vi "Nick FP.vi"() -> ()   [LabVIEW 2013]
uses:
  cPAS/Interface/CRDS/Controls/Ringdown Xctl/Ringdown.xctl
  Reusable/CRDS/Data/Cell/extparam.ctl
  cPAS/UI/CRDS/Subject/CRD Subject.lvclass
  Timothy/File Observer/Tim File Observer.lvclass
  Reusable/Observer/Observer.lvclass/Observer.ctl
  Reusable/File IO/Class/File Observer.lvclass/File Observer.ctl
  Reusable/CRDS/Data/Main/CRDS Data.lvclass
  Reusable/Data/Data.lvclass
  Reusable/CRDS/Data/Cell/CRDS Cell Data.lvclass/CRDS Cell Data.ctl
  Reusable/Observer/Data Subject.lvclass/Data Subject.ctl
  Reusable/Observer/Accessors/Read Observer Refs.vi
  Reusable/Observer/Accessors/Read DVR.vi
  Reusable/CRDS/Data/Cell/Read extParam.vi
  Reusable/File IO/Class/Write Write.vi
  Reusable/Observer/Write Data Queue.vi
  Reusable/File IO/Class/Accessors/Write File Ext.vi
  Reusable/File IO/Class/Accessors/Write File Prefix.vi
  Reusable/File IO/Class/Accessors/Write Max Size.vi
  Reusable/File IO/Class/Accessors/Write Top Data Path.vi
  <vilib>/addons/Digital Filter Design/Process.llb/DFD Filtering (Array).vi
  Reusable/CRDS/Data/Main/Read CellData.vi
  Reusable/Data/Read measTime.vi
  Reusable/CRDS/Data/Cell/Read Ringdowns.vi
  Reusable/Observer/Data Subject.lvclass
  Reusable/File IO/Class/File Observer.lvclass
  Reusable/Observer/Observer.lvclass
  Reusable/CRDS/Data/Cell/CRDS Cell Data.lvclass
  <vilib>/addons/Digital Filter Design/NI_DigFilterLicensed.lvlib
panel:
  out "Waveform Graph":dbl[][](graph)
  out "Ext Data":T1[](array[typedef])
  out "tau":T2(graph)
  in  "Write?":bool
  in  "SamplesPerCycle":u16=100
  in  "PointsPerCycle":u16=1000
  out "Time":timestamp format="%<%H:%M:%S%3u>T"
  out "Ringdown":i16[][][](xcontrol)
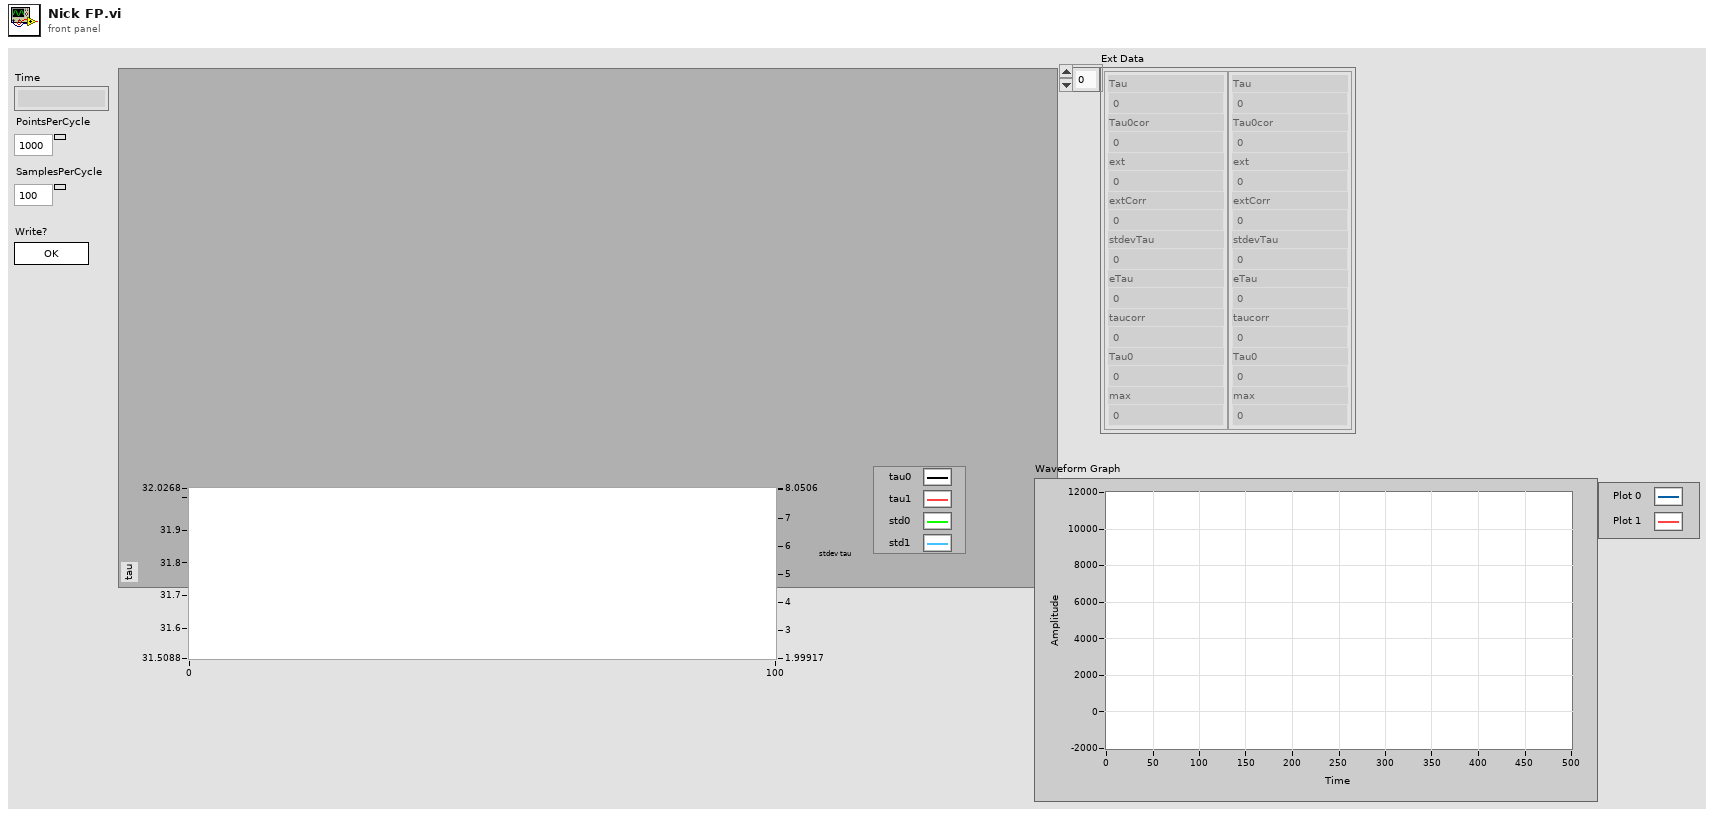
[diagram p1: front panel]
types:
  T1 = typedef "extparam.ctl" = cluster{"Tau":sgl, "Tau0cor":sgl, "ext":sgl, "extCorr":sgl, "stdevTau":sgl, "eTau":sgl, "taucorr":sgl, "Tau0":sgl, "max":sgl}
  T2 = cluster{"Tau":sgl, "Tau":sgl, "stdevTau":sgl, "stdevTau":sgl}
  T3 = typedef "NI_DigFilterLicensed.lvlib/DFD Filter Obj.ctl" = cluster{"mSRate_Fs":dbl, "mSRate_Version":string, "mSRate_Comments":string, "mSRate_OrgCoef":T4, "mSRate_CurCoef":T4, "mSRate_Quantized?":bool, "mSRate_QCoef":T4, "mSRate_QSettings":T6[], "mSRate_Order":i32, "mSRate_Scaling":cluster{"mSRate_ScaleByPowerOf2?":bool, "mSRate_ScaleType":T8}}
  T4 = typedef "NI_DigFilterLicensed.lvlib/DFD Filter Coef.ctl" = cluster{"type":T5, "gain":dbl, "coef a (k)":dbl[], "coef b (v)":dbl[]}
  T5 = typedef "NI_DigFilterLicensed.lvlib/DFD Filter Structure Type Selector.ctl" = enum16{"Undefined", "FIR Direct Form", "FIR Direct Form Transposed", "FIR Symmetric", "FIR Antisymmetric", "IIR Direct Form I", "IIR Direct Form I Transposed", "IIR Direct Form II", "IIR Direct Form II Transposed", "IIR Cascaded Second Order Sections Form I", "IIR Cascaded Second Order Sections Form I Transposed", "IIR Cascaded Second Order Sections Form II", "IIR Cascaded Second Order Sections Form II Transposed", "Lattice Allpass (basic sections)", "Lattice Allpass (one multiplier sections)", "Lattice Allpass (normalized sections)", "Lattice AR (basic sections)", "Lattice AR (one multiplier sections)", "Lattice AR (normalized sections)", "Lattice MA (minimum phase)", "Lattice MA (maximum phase)", "Lattice ARMA (basic sections)", "Lattice ARMA (one multiplier sections)", "Lattice ARMA (normalized sections)"}
  T6 = typedef "NI_DigFilterLicensed.lvlib/dfd_Internal Quantization Settings.ctl" = cluster{"source":T7, "wl":i16, "iwl":i16, "overflow mode":enum16{"Saturation", "Wrap"}, "rounding mode":enum16{"Nearest", "Truncation"}, "signed?":bool}
  T7 = typedef "NI_DigFilterLicensed.lvlib/dfd_Internal Quantization Srcs.ctl" = u16
  T8 = typedef "NI_DigFilterLicensed.lvlib/DFD Coef Norm Type.ctl" = enum16{"No Norm", "Time Domain 1-Norm", "Time Domain 2-Norm", "Time Domain Inf-Norm"}
  T9 = cluster{sgl, sgl, "stdevTau":sgl, "stdevTau":sgl}
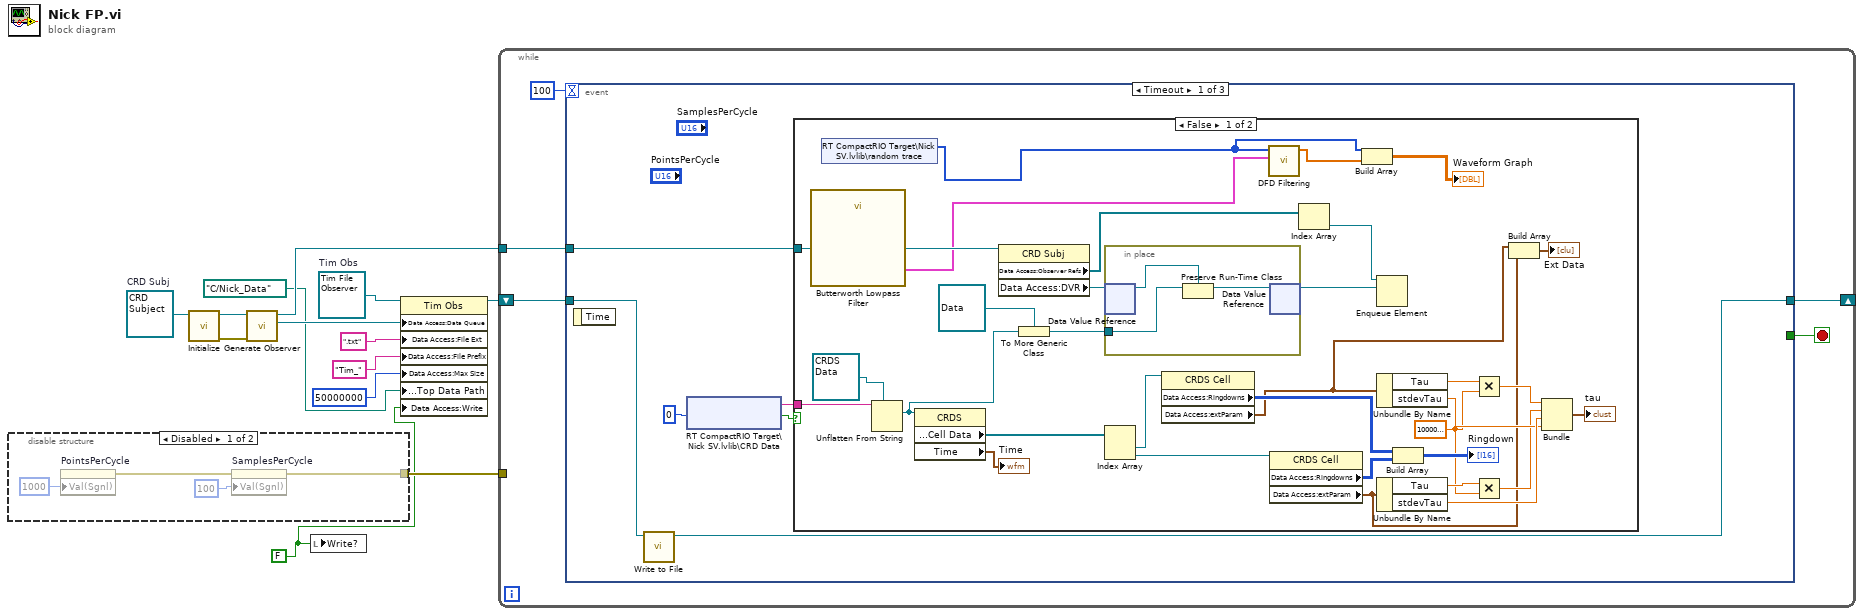
[diagram p0: block diagram]
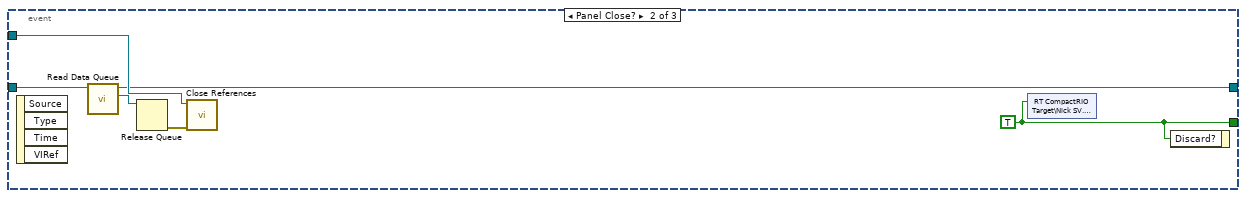
[diagram p4: hidden frame]
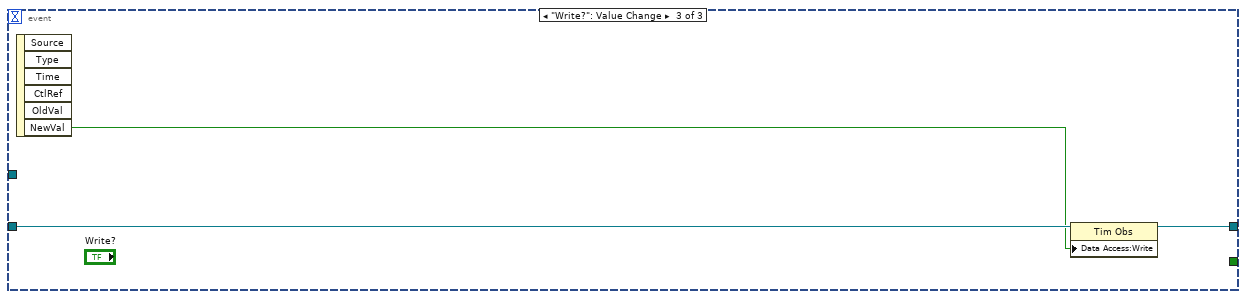
[diagram p5: hidden frame]
diagram:
  w2 = refnum<class "Tim File Observer.lvclass"> refnum  # Tim Obs
  w1 = FALSE ("Write")
  w12 = refnum<class "CRD Subject.lvclass"> refnum  # CRD Subj
  n1 = disable-structure shown="Disabled" {
    disable-tunnel: [w14 _] -> w13
    frame Disabled {
      n2 = property on="PointsPerCycle" class="DigNum (strict)"("Val(Sgnl)"=u16 1000 ("Value (Signaling)")) -> (error out=w15:errorcluster)  [unwired: 2 in, 1 out]
      n3 = property on="SamplesPerCycle" class="DigNum (strict)"(error in=w15, "Val(Sgnl)"=u16 100 ("Value (Signaling)")) -> (error out=w14:errorcluster)  [unwired: 1 in, 1 out]
    }
    frame Enabled {
    }
  }
  n4 = call-dynamic "Initialize.vi"("CRD Subject in"=w12) -> ("error out"=w10:errorcluster, "CRD Subject out"=w11:refnum<class "CRD Subject.lvclass">)  [unwired: 8 in, 1 out]
  n5 = call "Generate Observer.vi"("error in"=w10, "Data Subject in"=w11) -> ("Observer"=w9:refnum<queue>, "Data Subject out"=w8:refnum<class "CRD Subject.lvclass">)  [unwired: 7 in, 1 out]
  n6 = local write "Write?"(w1) -> ()
  n7 = property class="Tim Obs"(reference=w2, "Data Access:Data Queue"=w9, "Data Access:File Ext"=".txt" ("File Ext"), "Data Access:File Prefix"="Tim_" ("File Prefix"), "Data Access:Max Size"=i64 50000000 ("Max Size"), "Data Access:Top Data Path"=path "C:/Nick_Data" ("Top Data Path"), "Data Access:Write"=w1) -> (reference out=w3:refnum<class "Tim File Observer.lvclass">)  [unwired: 1 in, 1 out]
  n8 = while {
    tunnel: w13 -> [_]
    tunnel: w8 -> [w20]
    shift-right: [w18] -> _
    shift-left: w3 -> [w19]
    stop <- w22 stop-if-true
    n9 = event shown="[0] Timeout" {
      selector: _ -> [_ _ _]
      dyn-events: _ -> [_ _ _]
      timeout: 100 -> [_ _ _]
      tunnel: [_ w69 _] -> w22
      tunnel: w20 -> [w25 w68 _]
      tunnel: w19 -> [w24 w67 w72]
      tunnel: [w23 w64 w70] -> w18
      event Timeout {
        n10 = event-data() -> ()  [unwired: 1 in, 1 out]
        n11 = call "Write to File.vi"("File Obs in"=w24) -> ("File Obs out"=w23:refnum<class "Tim File Observer.lvclass">)  [unwired: 9 in, 1 out]
        n12 = shared-variable "RT CompactRIO Target\\Nick SV.lvlib\\CRD Data"(0 ("ms timeout (0)")) -> (w28:string, w26:bool)  [unwired: 1 in, 1 out]
        n13 = case shown="False" w26 {
          tunnel: w28 -> [w60 _]
          tunnel: w25 -> [w53 _]
          frame False {
            w37 = sgl 1000000.0 ("y")
            n14 = call "Butterworth Lowpass Filter"() -> ("filter out"=w32:T3)  [unwired: 10 in, 1 out]
            n15 = shared-variable "RT CompactRIO Target\\Nick SV.lvlib\\random trace"() -> (w30:i16[])  [unwired: 1 in, 1 out]
            n16 = Unflatten From String(type=refnum<class "CRDS Data.lvclass"> refnum ("CRDS"), binary string=w60) -> (value=w50:refnum<class "CRDS Data.lvclass">)  [unwired: 3 in, 2 out]
            n17 = property class="CRDS"(reference=w50) -> ("Data Access:Cell Data"=w57:refnum<class "CRDS Cell Data.lvclass">[], "Time"=→"Time":timestamp)  [unwired: 1 in, 2 out]
            n18 = property class="CRD Subj"(reference=w53) -> ("Data Access:Observer Refs"=w52:refnum<queue>[], "Data Access:DVR"=w48:refnum<data-value>)  [unwired: 1 in, 2 out]
            n19 = To More Generic Class(target class=refnum<class "Data.lvclass"> refnum ("Base Data Class.lvlib:Data"), reference=w50) -> (generic class reference=w47:refnum<class "Data.lvclass">)
            n20 = in-place {
              in-place-border: w47 -> [w63]
              n21 = in-place-dvr #1(w48) -> (w62:refnum<class "Data.lvclass">)  [unwired: 1 out]
              n22 = Preserve Run-Time Class(object in=w63, 2:w62) -> (object out=w61:refnum<class "Data.lvclass">)  [unwired: 1 in, 1 out]
              n23 = in-place-dvr #1(w61) -> (w46:refnum<data-value>)  [unwired: 1 out]
            }
            n24 = Index Array(array=w57) -> (element #1=w58:refnum<class "CRDS Cell Data.lvclass">, element #2=w44:refnum<class "CRDS Cell Data.lvclass">)  [unwired: 2 in]
            n25 = property class="CRDS Cell"(reference=w58) -> ("Data Access:Ringdowns"=w55:i16[][], "Data Access:extParam"=w35:T1)  [unwired: 1 in, 2 out]
            n26 = call-poly <vilib>:"DFD Filtering.vi"("filter"=w32, "signal in"=w30) -> ("signal out"=w31:dbl[])  [unwired: 8 in, 1 out]
            n27 = property class="CRDS Cell"(reference=w44) -> ("Data Access:Ringdowns"=w43:i16[][], "Data Access:extParam"=w34:T1)  [unwired: 1 in, 2 out]
            n28 = Index Array(array=w52) -> (element=w51:refnum<queue>)  [unwired: 1 in]
            n29 = Build Array(w30, w31) -> (→"Waveform Graph":dbl[][])
            n30 = Enqueue Element(queue=w51, element=w46) -> ()  [unwired: 2 in, 3 out]
            n31 = Unbundle By Name(w35) -> ("Tau"=w38:sgl, "stdevTau"=w41:sgl)
            n32 = Unbundle By Name(w34) -> ("Tau"=w40:sgl, "stdevTau"=w42:sgl)
            n33 = Build Array(w55, w43) -> (→"Ringdown":i16[][][])
            n34 = Multiply(x=w38, y=w37) -> (x*y=w36:sgl)
            n35 = Multiply(x=w40, y=w37) -> (x*y=w39:sgl)
            n36 = Build Array(w35, w34) -> (→"Ext Data":T1[])
            n37 = Bundle(w36, w39, "stdevTau"=w42, "stdevTau"=w41) -> (→"tau":T9)  [unwired: 1 in]
          }
          frame True {
          }
        }
      }
      event Panel Close? {
        w69 = TRUE ("Discard?")
        n38 = event-data() -> ()  [unwired: 1 in, 4 out]
        n39 = call "Read Data Queue.vi"("Observer in"=w67) -> ("Data Queue"=w66:refnum<queue>, "Observer out"=w64:refnum<class "Tim File Observer.lvclass">)  [unwired: 8 in, 1 out]
        n40 = Release Queue(queue=w66) -> (error out=w65:errorcluster)  [unwired: 2 in, 2 out]
        n41 = call "Close References.vi"("error in"=w65, "Data Subject in"=w68) -> ()  [unwired: 8 in, 2 out]
        n42 = shared-variable "RT CompactRIO Target\\Nick SV.lvlib\\Stop"(w69) -> ()  [unwired: 1 in, 1 out]
        n43 = event-data("Discard?"=w69) -> ()  [unwired: 1 in, 1 out]
      }
      event "Write?": Value Change {
        n44 = event-data() -> ("NewVal"=w71:bool)  [unwired: 1 in, 5 out]
        n45 = property class="Tim Obs"(reference=w72, "Data Access:Write"=w71) -> (reference out=w70:refnum<class "Tim File Observer.lvclass">)  [unwired: 1 in, 1 out]
      }
    }
  }
